vi "New IO Node.vi"(7 "Current Bus Path":path=path "D:/Documents/Projects/SPIAPI/IOEngineCode/Initialize Node Resources.vi", 8 "error in":errorcluster, 9 "Device Information":T1={"Number of Channels"=1, "Device Alias"="", "Icon Text"={"Line 1 text"="Bus", "Line 2 text"="Dev", "Line 3 text"="Ch", "Line 4 text"=""}}, 10 "Values for Naming":T3={"Bus Number"=1, "Device Number"=1, "Channel Number"=1} {"Channel Number" min=1 step=1; "Device Number" min=1 step=1; "Bus Number" min=1 step=1}, 11 "Virtual Folder":refnum<vi>) -> (0 "error out":errorcluster, 2 "Path to New Node":path, 3 "Path to IO Node":path=path "D:/Documents/Projects/SPIAPI/IOEngineCode/Initialize Node Resources.vi")   [LabVIEW 2014, in "SPI Engine Scripting.lvlib"]
doc: "Creates IO Node VI and adds it to a virtual folder and library."
uses:
  SPI Engine Scripting.lvlib
  State Machine/Controls/Values for Naming.ctl
  State Machine/Controls/Device Information.ctl
  <vilib>/LabVIEW Icon API/API_Text.ctl
  <vilib>/LabVIEW Icon API/LabVIEW Icon API.lvlib
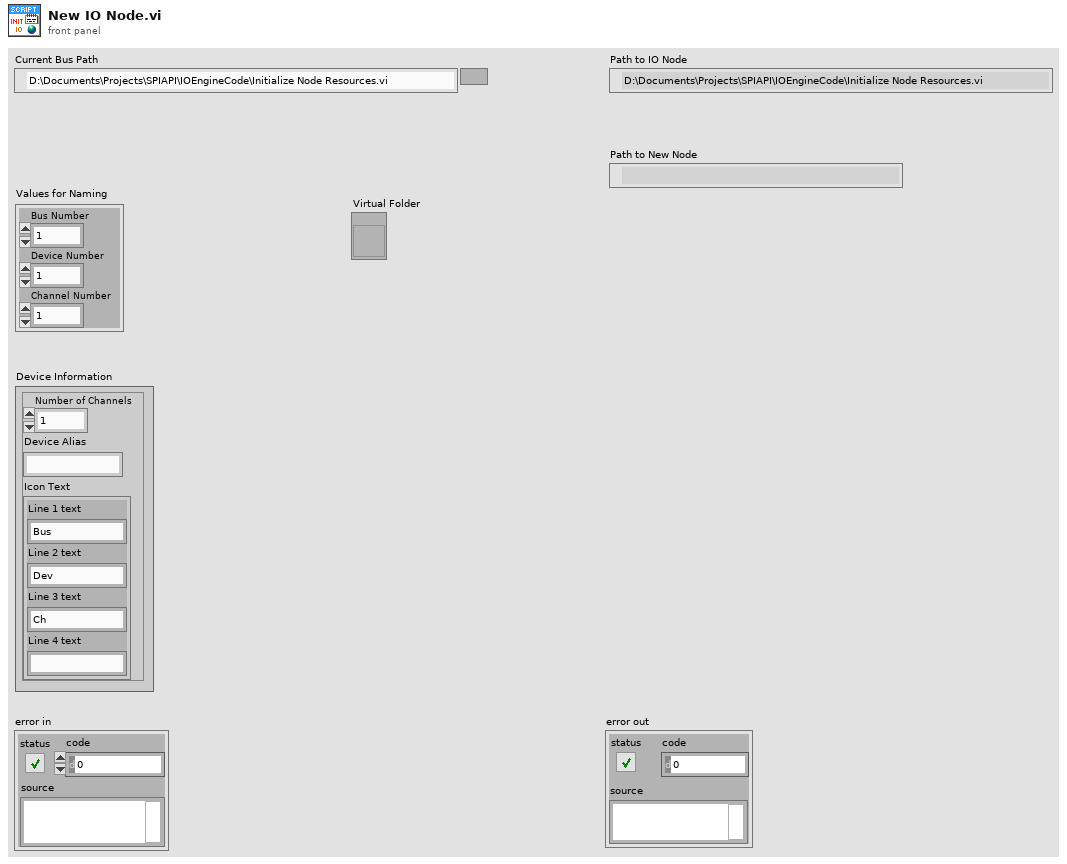
[diagram p1: front panel]
types:
  T1 = typedef "Device Information.ctl" = cluster{"Number of Channels":i32, "Device Alias":string, "Icon Text":T2}
  T2 = typedef "LabVIEW Icon API.lvlib/API_Text.ctl" = cluster{"Line 1 text":string, "Line 2 text":string, "Line 3 text":string, "Line 4 text":string}
  T3 = typedef "SPI Engine Scripting.lvlib/Values for Naming.ctl" = cluster{"Bus Number":i32, "Device Number":i32, "Channel Number":i32}
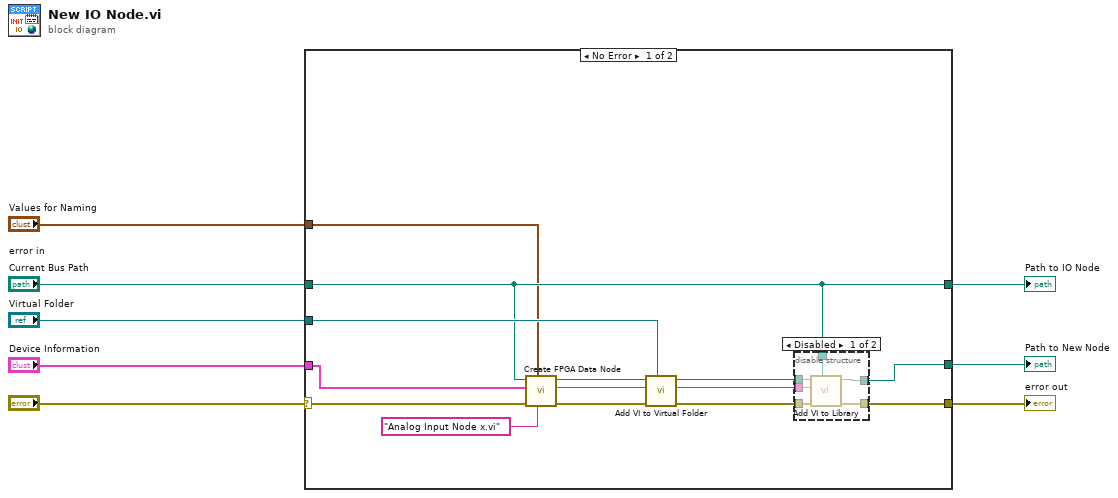
[diagram p0: block diagram]
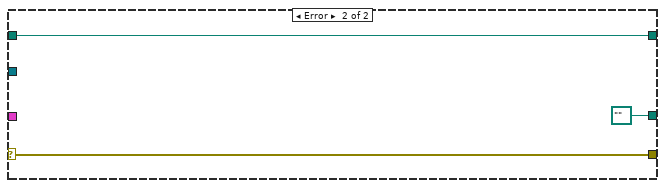
[diagram p3: hidden frame]
diagram:
  n1 = case shown="No Error" "error in" {
    selector: "error in" -> [w22 w34]
    tunnel: "Current Bus Path" -> [w14 w33]
    tunnel: [w13 w34] -> w6
    tunnel: [w14 w33] -> w5
    tunnel: "Virtual Folder" -> [w18 _]
    tunnel: "Values for Naming" -> [w10 _]
    tunnel: [w12 path "" ("Path to VI")] -> w2
    tunnel: "Device Information" -> [w9 _]
    frame No Error {
      n2 = call "Create FPGA Data Node.vi"("Path to Analog Node Template"="Analog Input Node x.vi", "Values for Naming"=w10, "error in"=w22, "Device Information"=w9, "Path to IO Node"=w14) -> ("error out"=w21:errorcluster, "IO Node Name"=w20:string, "Path to new IO Node"=w19:path)  [unwired: 4 in]
      n3 = call "Add VI to Virtual Folder.vi"("Virtual Folder"=w18, "error in"=w21, "VI Name"=w20, "Path to VI"=w19) -> ("error out"=w17:errorcluster, "VI Name"=w16:string, "Path to VI"=w15:path)  [unwired: 5 in]
      n4 = disable-structure shown="Disabled" {
        disable-tunnel: w17 -> [w29 w30]
        disable-tunnel: w16 -> [w28 _]
        disable-tunnel: w15 -> [w27 w31]
        disable-tunnel: w14 -> [w26 _]
        disable-tunnel: [w25 w30] -> w13
        disable-tunnel: [w24 w31] -> w12
        frame Disabled {
          n5 = call "Add VI to Library.vi"("Current Bus Path"=w26, "error in"=w29, "VI Name"=w28, "Path to new VI"=w27) -> ("error out"=w25:errorcluster, "Path to new IO Node"=w24:path, "Bus Number"=w23:i32)  [unwired: 5 in]
        }
        frame Enabled {
        }
      }
    }
    frame Error {
    }
  }
  "error out" <- w6
  "Path to IO Node" <- w5
  "Path to New Node" <- w2
